vi "Main Page.vi"(8 "error in (no error)":errorcluster, 11 "Node Ptr":T1 format="%.0x") -> (0 "error out":errorcluster)   [LabVIEW 2015, in "Engine Simulation Toolkit System Explorer.lvlib"]
uses:
  Engine Simulation Toolkit System Explorer.lvlib
  <vilib>/NI Veristand/Custom Device API/Custom Device Item Ref.ctl
  Listbox State.ctl
  Main Page refnums.ctl
  Shared/Properties.vi
  <vilib>/NI Veristand/Custom Device API/Set Item Property (Boolean).vi
  <vilib>/NI Veristand/Custom Device API/Get Item Property (I32).vi
  <vilib>/NI Veristand/Custom Device API/Get Item Property (String Array).vi
  <vilib>/NI Veristand/Custom Device API/Get Item Property (Dependent File).vi
  <vilib>/NI Veristand/Custom Device API/Get Item Property (String).vi
  <vilib>/NI Veristand/Custom Device API/Set Item Property (I32).vi
  Shared/Constants and GUIDs.vi
  <userlib>/_OpenG.lib/array/array.llb/Delete Elements from 2D Array (String)__ogtk.vi
  <userlib>/_OpenG.lib/array/array.llb/Index 2D Array Elements (String)__ogtk.vi
  <vilib>/NI VeriStand/Custom Device API/Custom Device API.lvlib
  Shared/Engine Simulation Toolkit Shared.lvlib
  <vilib>/NI VeriStand/Custom Device Tools/Custom Device Utility Library/Custom Device Utility Library.lvlib
panel:
  in  "Reload bitfile":bool
  in  "Set master":bool
  in  "Remove bitfile":bool
  in  "Add bitfile":bool
  in  "Bitfile listbox":i32[](listbox) caption="Available APUs"
  in  "Header 3":cluster{"Section Name":string}={"Section Name"="Bitfile Selection"}
  in  "Remove APU":bool
  in  "Add APU":bool
  in  "APU listbox":i32[](listbox) caption="Available APUs"
  in  "Header 2":cluster{"Section Name":string}={"Section Name"="Available APUs"}
  in  "CPU":i32=-2
  in  "Rate decimation":i32=1 min=1
  in  "Execution priority":enum16{"Low", "Medium", "High"}(ring)=enum."Medium"
  out "CD Version":string caption="Custom device version"
  in  "Header":cluster{"Section Name":string}={"Section Name"="Engine Simulation Toolkit Settings"}
  in  "Name":string
  # "(-2: automatic)"
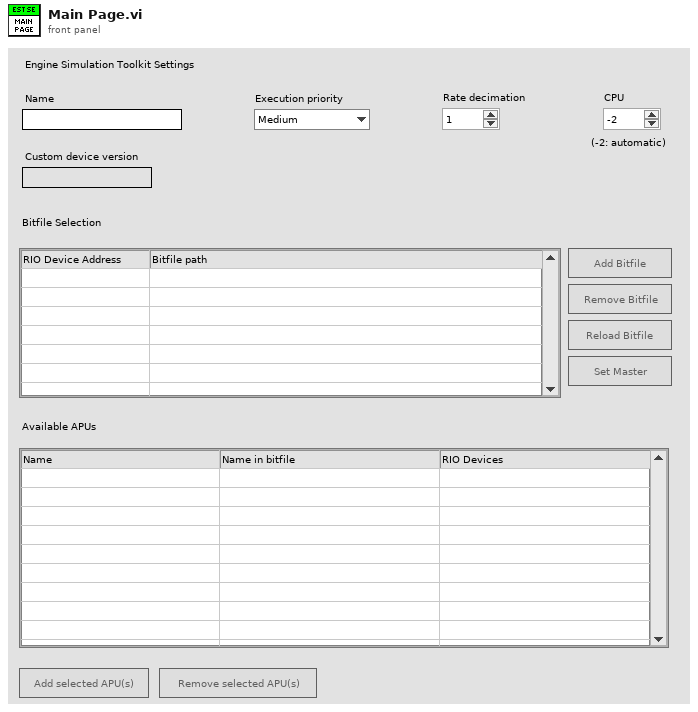
[diagram p1: front panel]
types:
  T1 = typedef "Custom Device API.lvlib/Custom Device Item Ref.ctl" = u64
  T2 = typedef "Engine Simulation Toolkit System Explorer.lvlib/Main Page refnums.ctl" = cluster{"Bitfile control refnums":cluster{"Add bitfile":refnum<vi>, "Remove bitfile":refnum<vi>, "Reload bitfile":refnum<vi>, "Set master":refnum<vi>, "Bitfile listbox":refnum<vi>}, "APU control refnums":cluster{"Add APU":refnum<vi>, "Remove APU":refnum<vi>, "APU listbox":refnum<vi>}}
  T3 = typedef "Engine Simulation Toolkit System Explorer.lvlib/Listbox State.ctl" = cluster{"listbox text":string[][], "not present item indexes":i32[], "selected values":i32[]}
  T4 = typedef "Custom Device API.lvlib/Custom Device Timed Loop Priority.ctl" = enum32{"Low", "Medium", "High"}
  T5 = typedef "Custom Device API.lvlib/Custom Device Item Info.ctl" = cluster{"Name":string, "Is Channel":bool, "GUID":string, "Is Waveform":bool}
  T6 = typedef "Custom Device API.lvlib/Custom Device Commands.ctl" = enum16{"Default", "Item renamed", "Shutdown", "Dynamic button pressed"}
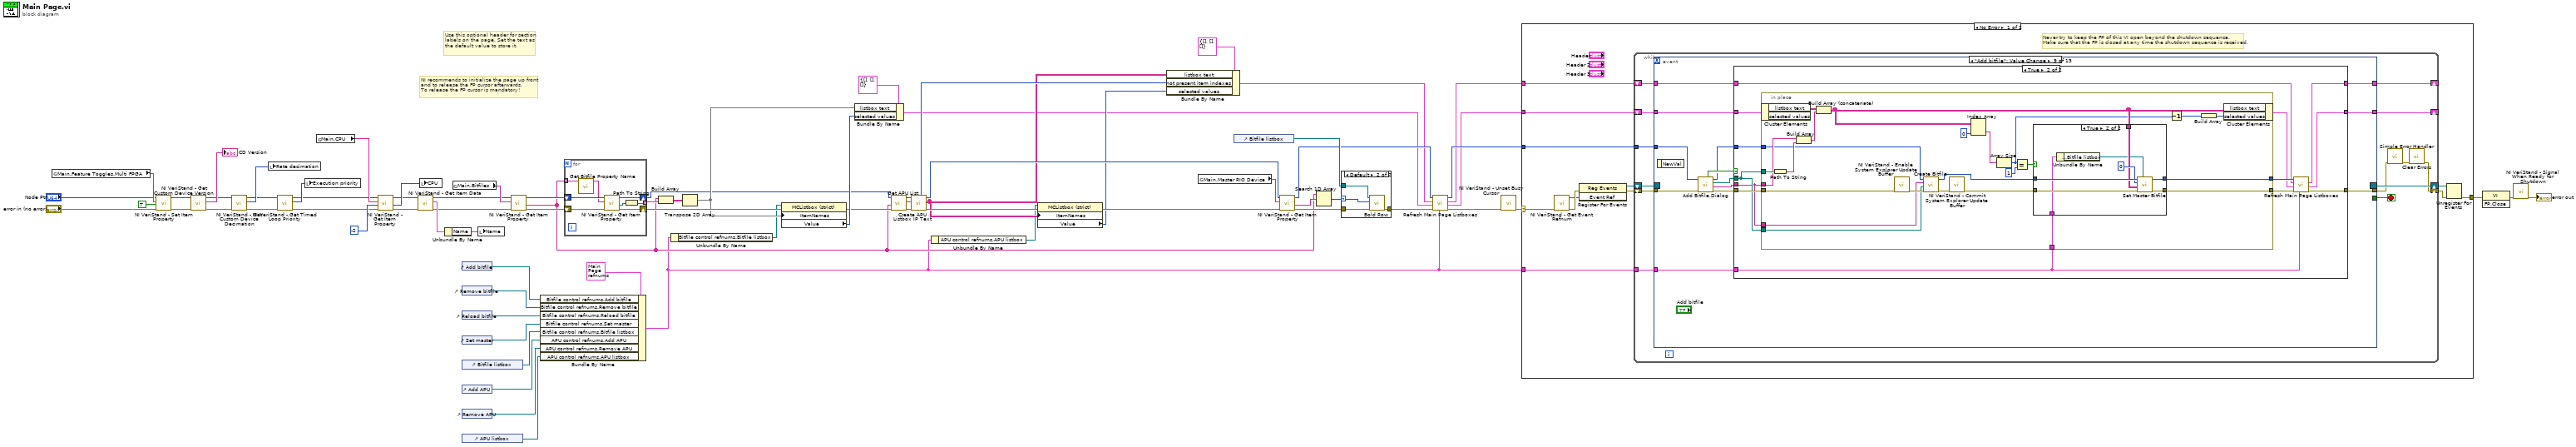
[diagram p0: block diagram]
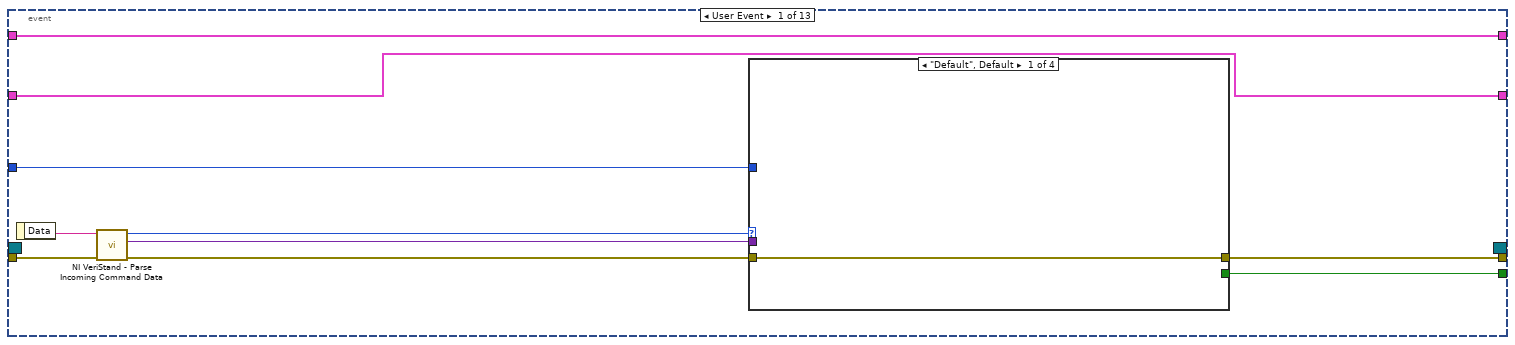
[diagram p3: hidden frame]
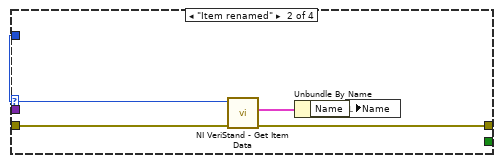
[diagram p4: hidden frame]
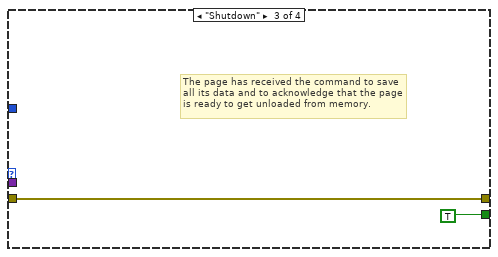
[diagram p5: hidden frame]
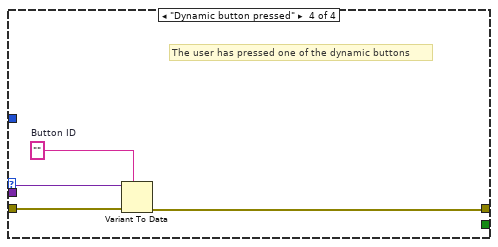
[diagram p6: hidden frame]
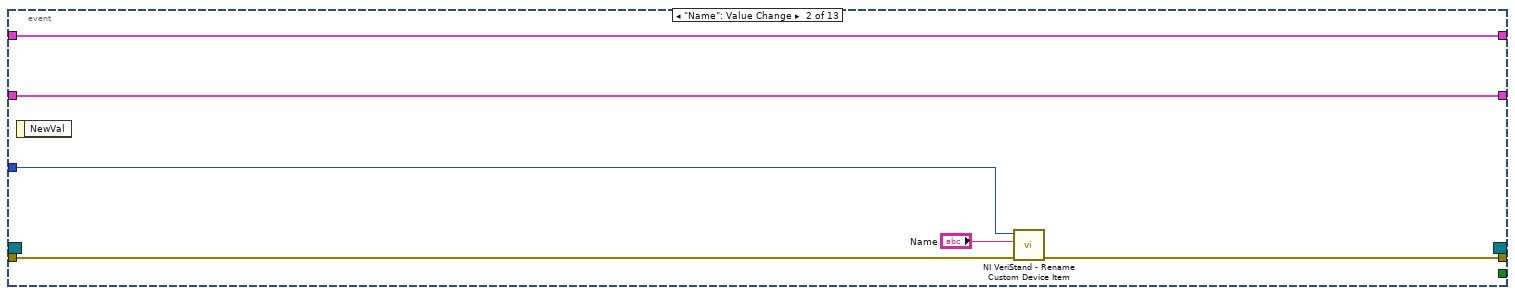
[diagram p7: hidden frame]
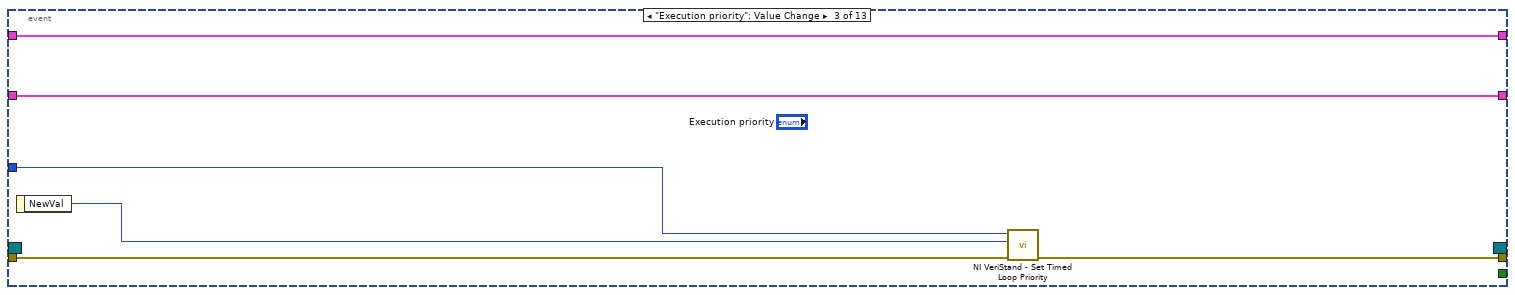
[diagram p8: hidden frame]
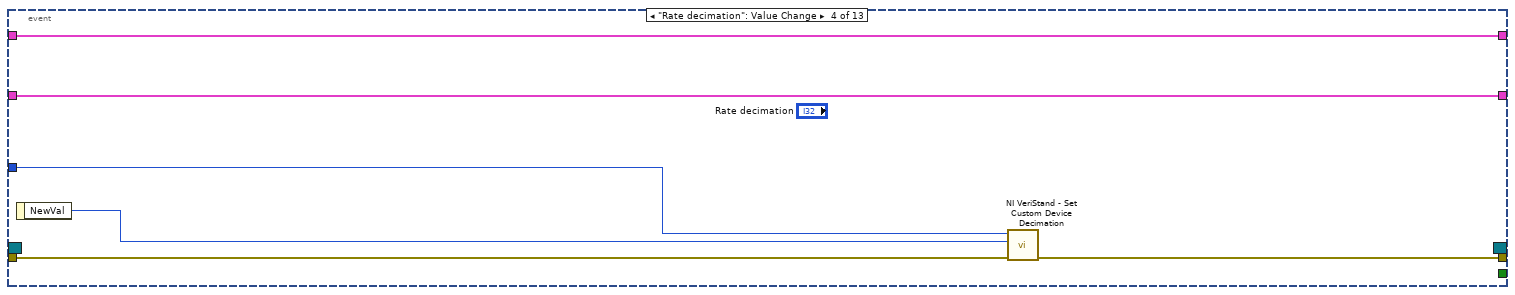
[diagram p9: hidden frame]
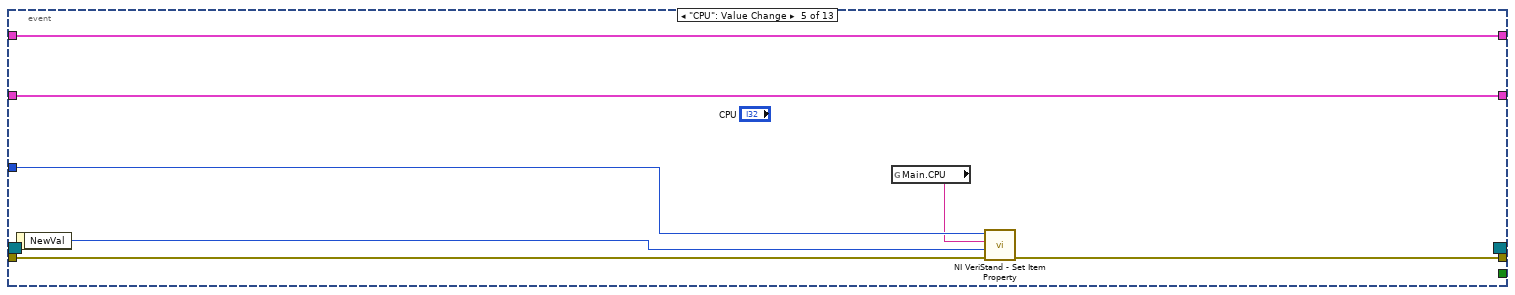
[diagram p10: hidden frame]
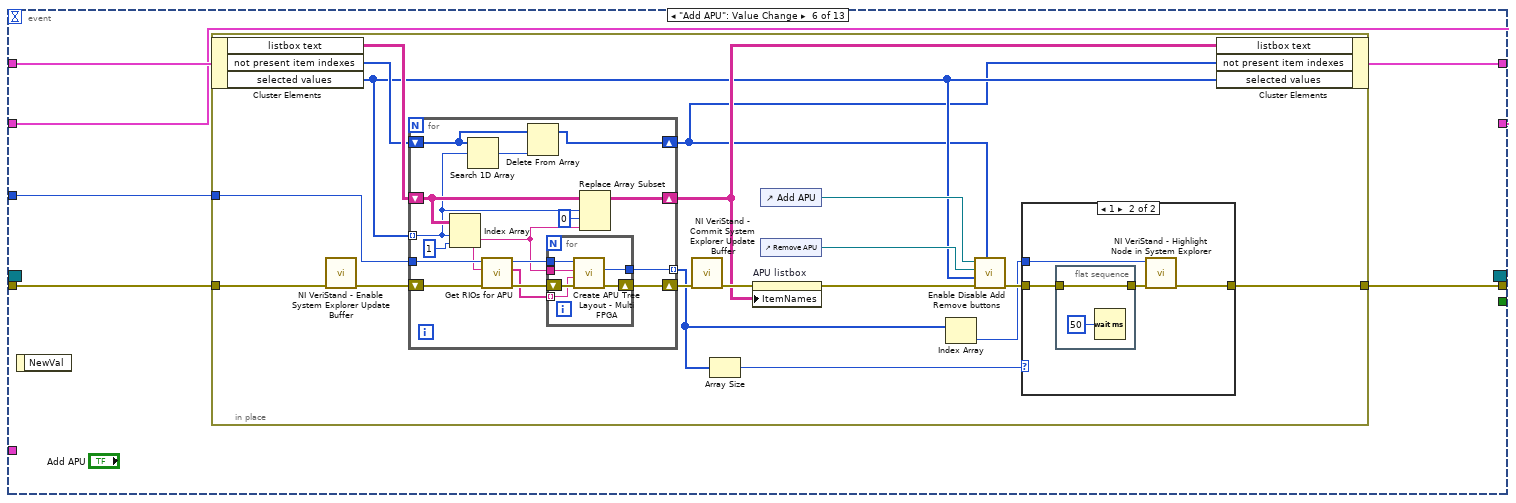
[diagram p11: hidden frame]
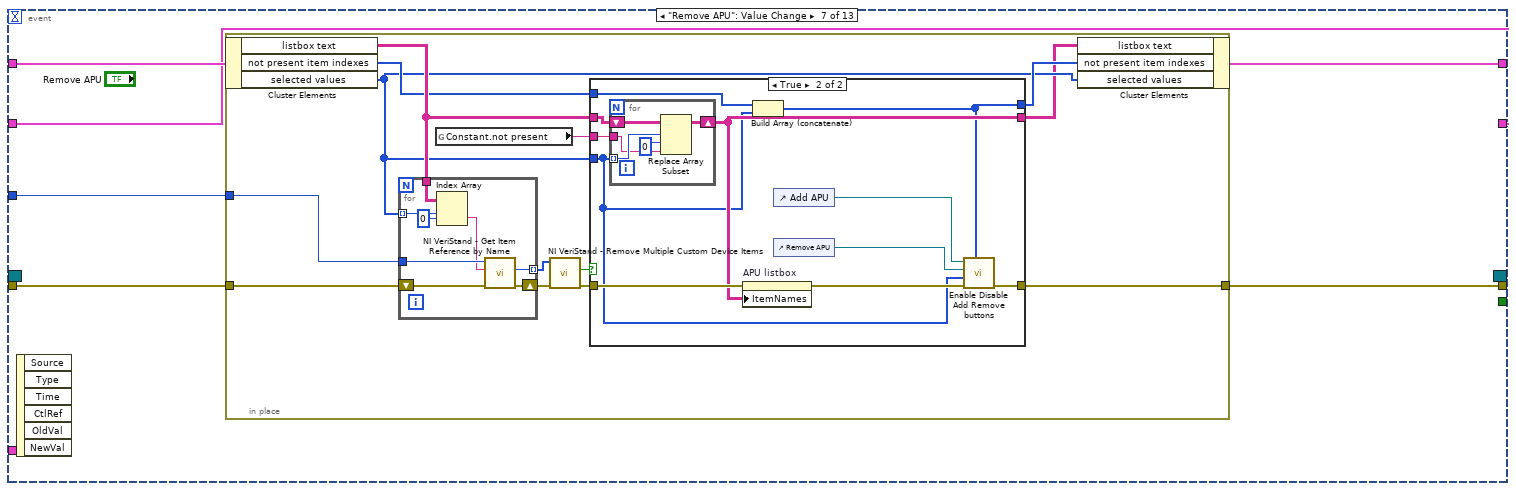
[diagram p13: hidden frame]
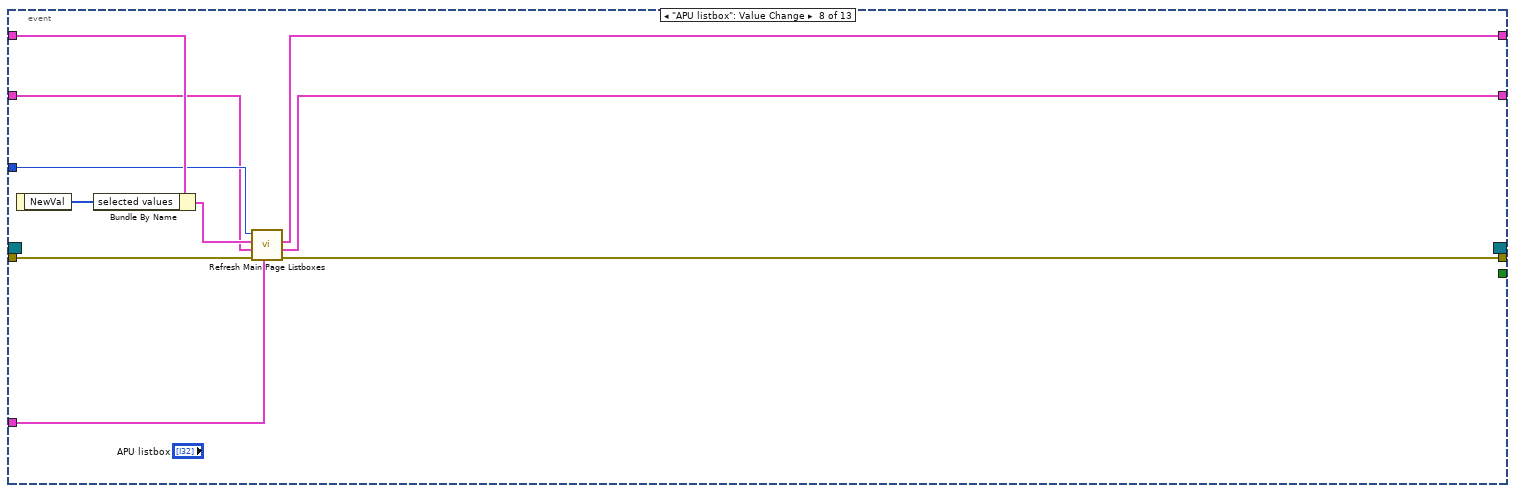
[diagram p15: hidden frame]
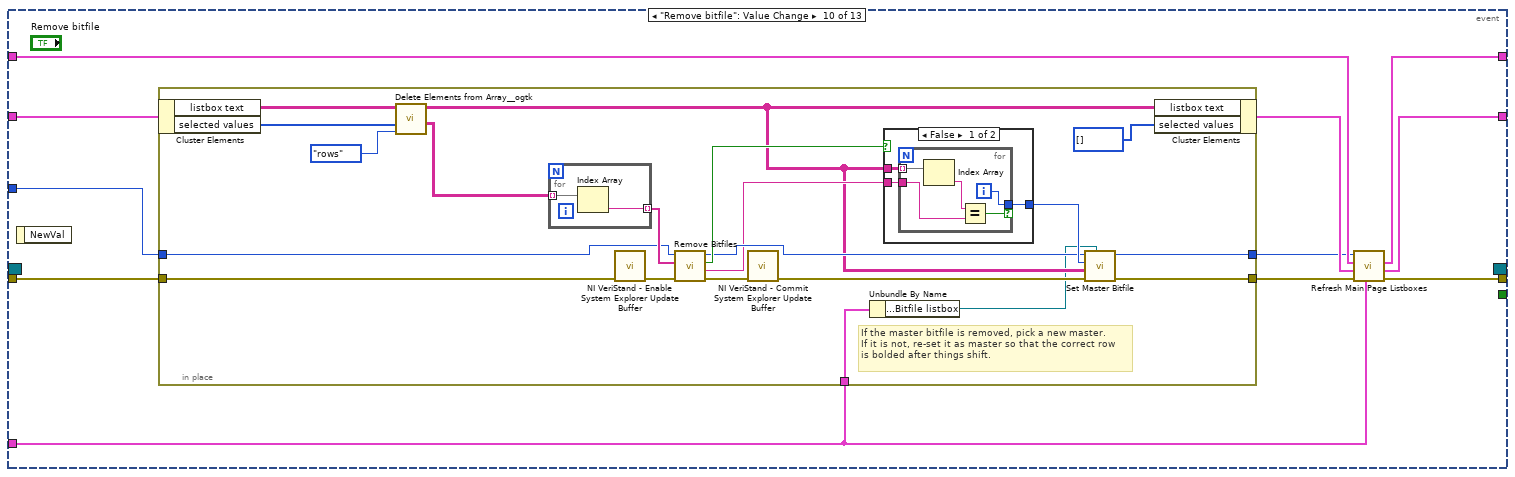
[diagram p18: hidden frame]
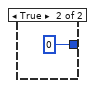
[diagram p19: hidden frame]
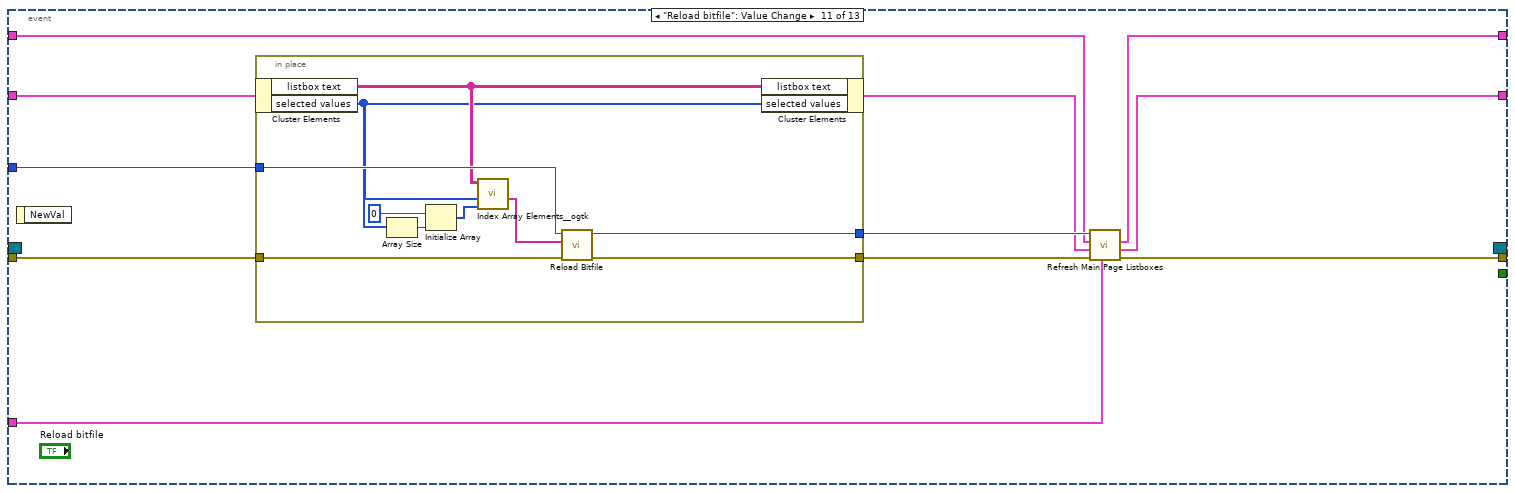
[diagram p20: hidden frame]
diagram:
  # "Use this optional header for section labels on the page. Set the text as the default value to store it."
  # "NI recommends to initialize the page up front\nand to release the FP cursor afterwards.\nTo release the FP cursor is mandatory!"
  n1 = global read "Properties.vi" "Main.Feature Toggles.Multi FPGA"() -> (w26:string)
  n2 = call-poly <vilib>:"NI VeriStand - Set Item Property.vi"("error in (no error)"="error in (no error)", "Value"=TRUE, "Property Name"=w26, "Item Ref in"="Node Ptr") -> ("error out"=w24:errorcluster, "Item Ref out"=w23:T1)  [unwired: 5 in, 1 out]
  n3 = call <vilib>:"NI VeriStand - Get Custom Device Version.vi"("error in (no error)"=w24, "Device Ref in"=w23) -> ("error out"=w69:errorcluster, "Value"=→"CD Version":string, "Device Ref out"=w66:T1)  [unwired: 7 in]
  n4 = call <vilib>:"NI VeriStand - Get Custom Device Decimation.vi"("error in (no error)"=w69, "Device Ref in"=w66) -> ("error out"=w67:errorcluster, "Decimation"=w65:i32, "Device Ref out"=w64:T1)  [unwired: 7 in]
  n5 = local write "Rate decimation"(w65) -> ()
  n6 = call <vilib>:"NI VeriStand - Get Timed Loop Priority.vi"("error in (no error)"=w67, "Device Ref in"=w64) -> ("error out"=w29:errorcluster, "Priority"=w63:T4, "Device Ref out"=w30:T1)  [unwired: 7 in]
  n7 = local write "Execution priority"(w63) -> ()
  n8 = global read "Properties.vi" "Main.CPU"() -> (w62:string)
  n9 = call-poly <vilib>:"NI VeriStand - Get Item Property.vi"("error in (no error)"=w29, "Default Value"=-2, "Property Name"=w62, "Item Ref in"=w30) -> ("error out"=w32:errorcluster, "Value"=w60:i32, "Item Ref out"=w33:T1)  [unwired: 4 in, 1 out]
  n10 = call <vilib>:"NI VeriStand - Get Item Data.vi"("error in (no error)"=w32, "Item Ref in"=w33) -> ("error out"=w38:errorcluster, "Item Info"=w71:T5, "Item Ref out"=w39:T1)  [unwired: 7 out]
  n11 = local write "CPU"(w60) -> ()
  n12 = Unbundle By Name(w71) -> ("Name"=w70:string)
  n13 = global read "Properties.vi" "Main.Bitfiles"() -> (w51:string)
  n14 = control-ref of="Add bitfile"() -> (w19:refnum<vi>)
  n15 = control-ref of="Remove bitfile"() -> (w18:refnum<vi>)
  n16 = control-ref of="Reload bitfile"() -> (w17:refnum<vi>)
  n17 = control-ref of="Set master"() -> (w16:refnum<vi>)
  n18 = control-ref of="Bitfile listbox"() -> (w13:refnum<vi>)
  n19 = control-ref of="Add APU"() -> (w15:refnum<vi>)
  n20 = control-ref of="Remove APU"() -> (w14:refnum<vi>)
  n21 = control-ref of="APU listbox"() -> (w12:refnum<vi>)
  n22 = local write "Name"(w70) -> ()
  n23 = call-poly <vilib>:"NI VeriStand - Get Item Property.vi"("error in (no error)"=w38, "Property Name"=w51, "Item Ref in"=w39) -> ("error out"=w50:errorcluster, "Value"=w31:string[], "Item Ref out"=w48:T1)  [unwired: 5 in, 1 out]
  n24 = Bundle By Name(cluster=T2 {"Bitfile control refnums"={"Add bitfile"=refnum, "Remove bitfile"=refnum, "Reload bitfile"=refnum, "Set master"=refnum, "Bitfile listbox"=refnum}, "APU control refnums"={"Add APU"=refnum, "Remove APU"=refnum, "APU listbox"=refnum}} ("Main Page refnums"), "Bitfile control refnums.Add bitfile"=w19, "Bitfile control refnums.Remove bitfile"=w18, "Bitfile control refnums.Reload bitfile"=w17, "Bitfile control refnums.Set master"=w16, "Bitfile control refnums.Bitfile listbox"=w13, "APU control refnums.Add APU"=w15, "APU control refnums.Remove APU"=w14, "APU control refnums.APU listbox"=w12) -> (w1:T2)
  n25 = for {
    shift-right: [w82] -> w49
    shift-left: w50 -> [w83]
    tunnel: [w78] -> w47 mode=indexing
    shift-right: [w80] -> w36
    shift-left: w48 -> [w81]
    tunnel: w31 -> [w76] mode=indexing
    n26 = call "Get Bitfile Property Name.vi"("RIO Device Address in"=w76) -> ("Bitfile Property Name"=w77:string)  [unwired: 10 in]
    n27 = call-poly <vilib>:"NI VeriStand - Get Item Property.vi"("error in (no error)"=w83, "Property Name"=w77, "Item Ref in"=w81) -> ("error out"=w82:errorcluster, "Path"=w79:path, "Item Ref out"=w80:T1)  [unwired: 4 in, 2 out]
    n28 = Path To String(path=w79) -> (string=w78:string)
  }
  n29 = Build Array(w31, w47) -> (w46:string[][])
  n30 = Unbundle By Name(w1) -> ("Bitfile control refnums.Bitfile listbox"=w11:refnum<vi>)
  n31 = Transpose 2D Array(2D array=w46) -> (transposed array=w45:string[][])
  n32 = property on="Property Node" class="MCListbox (strict)"(reference=w11, error in=w49, "ItemNames"=w45) -> (error out=w37:errorcluster, "Value"=w52:i32[])  [unwired: 1 out]
  n33 = Bundle By Name(cluster=T3 {"listbox text"=[], "not present item indexes"=[], "selected values"=[]} ("output cluster"), "listbox text"=w45, "selected values"=w52) -> (w3:T3)
  n34 = call "Get APU List.vi"("error in (no error)"=w37, "rio names"=w31, "Item Ref in"=w36) -> ("error out"=w59:errorcluster, "ips available"=w57:string[], "Item Ref out"=w58:T1)  [unwired: 6 in]
  n35 = call "Create APU Listbox IP Text.vi"("error in (no error)"=w59, "ips available"=w57, "Section Ref in"=w58) -> ("error out"=w56:errorcluster, "listbox text"=w28:string[][], "Section Ref out"=w35:T1, "not present item indexes"=w54:i32[])  [unwired: 5 in]
  n36 = Unbundle By Name(w1) -> ("APU control refnums.APU listbox"=w10:refnum<vi>)
  n37 = property on="Property Node" class="MCListbox (strict)"(reference=w10, error in=w56, "ItemNames"=w28) -> (error out=w55:errorcluster, "Value"=w27:i32[])  [unwired: 1 out]
  n38 = Bundle By Name(cluster=T3 {"listbox text"=[], "not present item indexes"=[], "selected values"=[]} ("output cluster"), "listbox text"=w28, "not present item indexes"=w54, "selected values"=w27) -> (w5:T3)
  n39 = global read "Properties.vi" "Main.Master RIO Device"() -> (w42:string)
  n40 = control-ref of="Bitfile listbox"() -> (w44:refnum<vi>)
  n41 = call-poly <vilib>:"NI VeriStand - Get Item Property.vi"("error in (no error)"=w55, "Property Name"=w42, "Item Ref in"=w35) -> ("error out"=w43:errorcluster, "Value"=w41:string, "Item Ref out"=w7:T1)  [unwired: 5 in, 1 out]
  n42 = Search 1D Array(1D array=w31, element=w41) -> (index of element=w40:i32)  [unwired: 1 in]
  n43 = case shown="Default" w40 {
    selector: w40 -> [_ w85]
    tunnel: w44 -> [_ w88]
    tunnel: [w84 w87] -> w9
    tunnel: w43 -> [w84 w86]
    frame -1 {
    }
    frame Default {
      n44 = call "Bold Row.vi"("error in (no error)"=w86, "Row (-2 : all)"=w85, "MulticolumnListbox in"=w88) -> ("error out"=w87:errorcluster)  [unwired: 7 in, 1 out]
    }
  }
  n45 = call "Refresh Main Page Listboxes.vi"("Main Page refnums"=w1, "error in (no error)"=w9, "bitfile listbox"=w3, "APU listbox"=w5, "Item Ref in"=w7) -> ("error out"=w8:errorcluster, "bitfile listbox out"=w2:T3, "APU listbox out"=w4:T3, "Item Ref out"=w6:T1)  [unwired: 3 in]
  n46 = call <vilib>:"NI VeriStand - Unset Busy Cursor.vi"("error in (no error)"=w8) -> ("error out"=w72:errorcluster)  [unwired: 10 out]
  n47 = case shown="No Error" w72 {
    selector: w72 -> [w92 w422]
    tunnel: [w97 w420] -> w75
    tunnel: w6 -> [w93 _]
    tunnel: w4 -> [w91 _]
    tunnel: w2 -> [w90 _]
    tunnel: w1 -> [w89 _]
    frame No Error {
      # "Never try to keep the FP of this VI open beyond the shutdown sequence.\nMake sure that the FP is closed at any time the shutdown sequence is received."
      n48 = call <vilib>:"NI VeriStand - Get Event Refnum.vi"("error in (no error)"=w92) -> ("error out"=w100:errorcluster, "Event Ref"=w96:refnum<user-event>)  [unwired: 9 out]
      n49 = register-events(error in=w100, w96) -> (reference out=w94:refnum<event-registration>, error out=w95:errorcluster)  [unwired: 1 in]
      n50 = while {
        tunnel: w93 -> [w109]
        shift-right: [w106] -> w98
        shift-left: w95 -> [w112]
        shift-right: [w113] -> w99
        shift-left: w94 -> [w111]
        shift-right: [w104] -> _
        shift-left: w91 -> [w105]
        shift-right: [w102] -> _
        shift-left: w90 -> [w103]
        tunnel: w89 -> [w101]
        stop <- w110 stop-if-true
        n51 = event shown="[8] \"Add bitfile\": Value Change" {
          selector: w111 -> [_ _ _ _ _ _ _ _ _ _ _ _ _]
          dyn-events: [_ _ _ _ _ _ _ _ _ _ _ _ _] -> w113
          timeout: _ -> [_ _ _ _ _ _ _ _ _ _ _ _ _]
          tunnel: w112 -> [w123 w141 w147 w153 w160 w166 w219 w267 w279 w343 w384 w409 w417]
          tunnel: [w119 _ _ _ _ _ _ _ _ _ _ _ _] -> w110
          tunnel: [w118 w140 w145 w151 w156 w165 w218 w266 w282 w335 w381 w398 w416] -> w108
          tunnel: w109 -> [w117 w139 w146 w152 w159 w164 w217 w265 w274 w341 w383 w404 w415]
          tunnel: w105 -> [w115 w137 w143 w149 w155 w163 w216 w268 w272 w339 w379 w402 w414]
          tunnel: [w115 w137 w143 w149 w155 w162 w215 w263 w271 w338 w378 w400 w411] -> w104
          tunnel: w103 -> [w114 w136 w142 w148 w154 w161 w214 w262 w281 w342 w385 w401 w419]
          tunnel: [w114 w136 w142 w148 w154 w161 w214 w261 w280 w337 w377 w399 w412] -> w102
          tunnel: w101 -> [_ _ _ _ _ _ _ w260 w270 w333 w375 w397 w410]
          event User Event {
            n52 = event-data() -> ("Data"=w122:string)  [unwired: 1 out]
            n53 = call <vilib>:"NI VeriStand - Parse Incoming Command Data.vi"("error in (no error)"=w123, "Incoming data"=w122) -> ("error out"=w121:errorcluster, "Outgoing data"=w116:variant, "Action"=w120:T6)  [unwired: 7 out]
            n54 = case shown="\"Default\", Default" w120 {
              tunnel: w121 -> [w124 w129 w130 w135]
              tunnel: [_ _ TRUE _] -> w119
              tunnel: [w124 w126 w130 w132] -> w118
              tunnel: w117 -> [_ w128 _ _]
              tunnel: w116 -> [_ _ _ w134]
              frame "Default", Default {
              }
              frame "Item renamed" {
                n55 = call <vilib>:"NI VeriStand - Get Item Data.vi"("error in (no error)"=w129, "Item Ref in"=w128) -> ("error out"=w126:errorcluster, "Item Info"=w127:T5)  [unwired: 8 out]
                n56 = Unbundle By Name(w127) -> ("Name"=w125:string)
                n57 = local write "Name"(w125) -> ()
              }
              frame "Shutdown" {
                # "The page has received the command to save all its data and to acknowledge that the page is ready to get unloaded from memory."
              }
              frame "Dynamic button pressed" {
                w133 = ""  # Button ID
                # "The user has pressed one of the dynamic buttons"
                n58 = Variant To Data(error in=w135, type=w133, Variant=w134) -> (error out=w132:errorcluster)  [unwired: 1 out]
              }
            }
          }
          event "Name": Value Change {
            n59 = event-data() -> ()  [unwired: 2 out]
            n60 = call <vilib>:"NI VeriStand - Rename Custom Device Item.vi"("error in (no error)"=w141, "New Name"="Name", "Item Ref in"=w139) -> ("error out"=w140:errorcluster)  [unwired: 1 in, 7 out]
          }
          event "Execution priority": Value Change {
            n61 = event-data() -> ("NewVal"=w144:enum16{"Low", "Medium", "High"})  [unwired: 1 out]
            n62 = call <vilib>:"NI VeriStand - Set Timed Loop Priority.vi"("error in (no error)"=w147, "Priority"=w144, "Device Ref in"=w146) -> ("error out"=w145:errorcluster)  [unwired: 7 in, 1 out]
          }
          event "Rate decimation": Value Change {
            n63 = event-data() -> ("NewVal"=w150:i32)  [unwired: 1 out]
            n64 = call <vilib>:"NI VeriStand - Set Custom Device Decimation.vi"("error in (no error)"=w153, "Decimation"=w150, "Device Ref in"=w152) -> ("error out"=w151:errorcluster)  [unwired: 7 in, 1 out]
          }
          event "CPU": Value Change {
            n65 = event-data() -> ("NewVal"=w158:i32)  [unwired: 1 out]
            n66 = global read "Properties.vi" "Main.CPU"() -> (w157:string)
            n67 = call-poly <vilib>:"NI VeriStand - Set Item Property.vi"("error in (no error)"=w160, "Value"=w158, "Property Name"=w157, "Item Ref in"=w159) -> ("error out"=w156:errorcluster)  [unwired: 5 in, 2 out]
          }
          event "Add APU": Value Change {
            n68 = event-data() -> ()  [unwired: 2 out]
            n69 = in-place {
              in-place-border: w166 -> [w174]
              in-place-border: [w173] -> w165
              in-place-border: w164 -> [w172]
              n70 = in-place-cluster #1(w163) -> ("listbox text"=w171:string[][], "not present item indexes"=w170:i32[], "selected values"=w168:i32[])
              n71 = call <vilib>:"NI VeriStand - Enable System Explorer Update Buffer.vi"("error in (no error)"=w174) -> ("error out"=w179:errorcluster)  [unwired: 10 in]
              n72 = for {
                tunnel: w172 -> [w195]
                shift-right: [w207] -> w184
                shift-left: w179 -> [w194]
                tunnel: w168 -> [w202] mode=indexing
                shift-right: [w204] -> w169
                shift-left: w171 -> [w205]
                shift-right: [w199] -> w167
                shift-left: w170 -> [w201]
                tunnel: [w198] -> w177 mode=indexing
                n73 = Index Array(array=w205, index (row)=w202, index (col)=1 ("disabled index (col)")) -> (element=w192:string)
                n74 = Search 1D Array(1D array=w201, element=w202) -> (index of element=w200:i32)  [unwired: 1 in]
                n75 = call "Get RIOs for APU.vi"("error in (no error)"=w194, "APU name"=w192, "Item Ref in"=w195) -> ("error out"=w197:errorcluster, "RIO Addresses"=w193:string[], "Item Ref out"=w196:T1)  [unwired: 6 in]
                n76 = Delete From Array(array=w201, index=w200) -> (array with subset deleted=w199:i32[])  [unwired: 1 in, 1 out]
                n77 = for {
                  tunnel: w192 -> [w212]
                  shift-right: [w213] -> w207
                  shift-left: w197 -> [w210]
                  tunnel: w193 -> [w208] mode=indexing
                  tunnel: w196 -> [w209]
                  tunnel: [w211] -> w198
                  n78 = call "Create APU Tree Layout - Multi FPGA.vi"("error in (no error)"=w210, "rio name"=w208, "engine name"=w212, "Section Ptr"=w209) -> ("error out"=w213:errorcluster, "APU ref"=w211:T1)  [unwired: 5 in, 1 out]
                }
                n79 = Replace Array Subset(array=w205, new element=w192, index (row)=w202, index (col)=0 ("disabled index (col)")) -> (w204:string[][])
              }
              n80 = call <vilib>:"NI VeriStand - Commit System Explorer Update Buffer.vi"("error in (no error)"=w184) -> ("error out"=w178:errorcluster)  [unwired: 10 in]
              n81 = Array Size(array=w177) -> (size(s)=w175:i32)
              n82 = property on="APU listbox" class="MCListbox (strict)"(error in=w178, "ItemNames"=w169) -> (error out=w183:errorcluster)  [unwired: 1 in, 1 out]
              n83 = control-ref of="Add APU"() -> (w181:refnum<vi>)
              n84 = control-ref of="Remove APU"() -> (w180:refnum<vi>)
              n85 = Index Array(array=w177) -> (element=w176:T1)  [unwired: 1 in]
              n86 = call "Enable Disable Add Remove buttons.vi"("not present item indexes"=w167, "error in (no error)"=w183, "selected items"=w168, "remove button"=w180, "add button"=w181) -> ("error out"=w182:errorcluster)  [unwired: 6 in]
              n87 = case shown="1" w175 {
                tunnel: w182 -> [w185 w186]
                tunnel: [w185 w189] -> w173
                tunnel: w176 -> [_ w188]
                frame Default {
                }
                frame 1 {
                  n88 = flat-sequence {
                    tunnel: [w190] -> w187
                    tunnel: w186 -> [w190]
                    frame #0 {
                      n89 = Wait (ms)(milliseconds to wait=u32 50) -> ()  [unwired: 1 out]
                    }
                  }
                  n90 = call <vilib>:"NI VeriStand - Highlight Node in System Explorer.vi"("error in (no error)"=w187, "Item Ref in"=w188) -> ("error out"=w189:errorcluster)  [unwired: 8 in, 1 out]
                }
              }
              n91 = in-place-cluster #1("listbox text"=w169, "not present item indexes"=w167, "selected values"=w168) -> (w162:T3)
            }
          }
          event "Remove APU": Value Change {
            n92 = event-data() -> ()  [unwired: 7 out]
            n93 = in-place {
              in-place-border: w219 -> [w227]
              in-place-border: [w226] -> w218
              in-place-border: w217 -> [w225]
              n94 = in-place-cluster #2(w216) -> ("listbox text"=w224:string[][], "not present item indexes"=w222:i32[], "selected values"=w221:i32[])
              n95 = for {
                tunnel: w221 -> [w258] mode=indexing
                tunnel: w224 -> [w259]
                tunnel: w225 -> [w255]
                tunnel: [w252] -> w231 mode=indexing
                shift-right: [w254] -> w232
                shift-left: w227 -> [w256]
                n96 = Index Array(array=w259, index (row)=w258, index (col)=0 ("disabled index (col)")) -> (element=w253:string)
                n97 = call <vilib>:"NI VeriStand - Get Item Reference by Name.vi"("error in (no error)"=w256, "Item Name"=w253, "Parent Ref in"=w255) -> ("error out"=w254:errorcluster, "Item Ref"=w252:T1)  [unwired: 5 in, 2 out]
              }
              n98 = global read "Constants and GUIDs.vi" "Constant.not present"() -> (w228:string)
              n99 = call <vilib>:"NI VeriStand - Remove Multiple Custom Device Items.vi"("error in (no error)"=w232, "Item Refs in"=w231) -> ("error out"=w230:errorcluster, "Deleted?"=w229:bool)  [unwired: 8 in]
              n100 = case shown="True" w229 {
                tunnel: [w234 w245] -> w226
                tunnel: w230 -> [w234 w242]
                tunnel: w221 -> [_ w237]
                tunnel: w224 -> [w235 w241]
                tunnel: w228 -> [_ w240]
                tunnel: [w235 w239] -> w220
                tunnel: w222 -> [w233 w238]
                tunnel: [w233 w236] -> w223
                frame False {
                }
                frame True {
                  n101 = for {
                    tunnel: w237 -> [w249] mode=indexing
                    shift-right: [w250] -> w239
                    shift-left: w241 -> [w251]
                    tunnel: w240 -> [w247]
                    n102 = Replace Array Subset(array=w251, new element=w247, index (row)=w249, index (col)=0 ("disabled index (col)")) -> (w250:string[][])
                  }
                  n103 = property on="APU listbox" class="MCListbox (strict)"(error in=w242, "ItemNames"=w239) -> (error out=w246:errorcluster)  [unwired: 1 in, 1 out]
                  n104 = Build Array (concatenate)(w238, w237) -> (w236:i32[])
                  n105 = control-ref of="Add APU"() -> (w244:refnum<vi>)
                  n106 = control-ref of="Remove APU"() -> (w243:refnum<vi>)
                  n107 = call "Enable Disable Add Remove buttons.vi"("not present item indexes"=w236, "error in (no error)"=w246, "selected items"=w237, "remove button"=w243, "add button"=w244) -> ("error out"=w245:errorcluster)  [unwired: 6 in]
                }
              }
              n108 = in-place-cluster #2("listbox text"=w220, "not present item indexes"=w223, "selected values"=w221) -> (w215:T3)
            }
          }
          event "APU listbox": Value Change {
            n109 = event-data() -> ("NewVal"=w269:i32[])  [unwired: 1 out]
            n110 = Bundle By Name(cluster=w268, "selected values"=w269) -> (w264:T3)
            n111 = call "Refresh Main Page Listboxes.vi"("Main Page refnums"=w260, "error in (no error)"=w267, "bitfile listbox"=w262, "APU listbox"=w264, "Item Ref in"=w265) -> ("error out"=w266:errorcluster, "bitfile listbox out"=w261:T3, "APU listbox out"=w263:T3)  [unwired: 3 in, 1 out]
          }
          event "Add bitfile": Value Change {
            n112 = event-data() -> ()  [unwired: 2 out]
            n113 = call "Add Bitfile Dialog.vi"("error in (no error)"=w279, "Item Ref in"=w274) -> ("error out"=w277:errorcluster, "RIO Device Address out"=w276:string, "Bitfile Path out"=w278:path, "Item Ref out"=w273:T1, "OK?"=w275:bool)  [unwired: 5 in]
            n114 = case shown="True" w275 {
              tunnel: w277 -> [w284 w298]
              tunnel: [w284 w292] -> w282
              tunnel: w281 -> [w285 w297]
              tunnel: [w285 w287] -> w280
              tunnel: w278 -> [_ w295]
              tunnel: w276 -> [_ w294]
              tunnel: w273 -> [_ w296]
              tunnel: w272 -> [w283 w290]
              tunnel: [w283 w289] -> w271
              tunnel: w270 -> [_ w286]
              frame False {
              }
              frame True {
                n115 = in-place {
                  in-place-border: [w312] -> w293
                  in-place-border: w295 -> [w320]
                  in-place-border: w294 -> [w318]
                  in-place-border: w298 -> [w317]
                  in-place-border: w296 -> [w308]
                  in-place-border: w295 -> [w304]
                  in-place-border: w294 -> [w305]
                  in-place-border: [w303] -> w291
                  in-place-border: w286 -> [w302]
                  n116 = in-place-cluster #3(w297) -> ("listbox text"=w322:string[][])  [unwired: 1 out]
                  n117 = Path To String(path=w320) -> (string=w319:string)
                  n118 = Build Array(w318, w319) -> (w321:string[])
                  n119 = Build Array (concatenate)(w322, w321) -> (w311:string[][])
                  n120 = call <vilib>:"NI VeriStand - Enable System Explorer Update Buffer.vi"("error in (no error)"=w317) -> ("error out"=w309:errorcluster)  [unwired: 10 in]
                  n121 = call "Create Bitfile.vi"("error in (no error)"=w309, "Bitfile Path in"=w304, "RIO Device Address in"=w305, "Item Ref in"=w308) -> ("error out"=w310:errorcluster, "Item Ref out"=w307:T1)  [unwired: 5 in, 1 out]
                  n122 = call <vilib>:"NI VeriStand - Commit System Explorer Update Buffer.vi"("error in (no error)"=w310) -> ("error out"=w306:errorcluster)  [unwired: 10 in]
                  n123 = Index Array(array=w311, index (col)=0 ("disabled index (col)")) -> (element=w313:string[])  [unwired: 1 in]
                  n124 = Array Size(array=w313) -> (size(s)=w300:i32)
                  n125 = Equal?(x=w300, y=1) -> (x = y?=w314:bool)
                  n126 = case shown="True" w314 {
                    tunnel: [w323 w330] -> w312
                    tunnel: w306 -> [w323 w329]
                    tunnel: w307 -> [w324 w332]
                    tunnel: [w324 w331] -> w303
                    tunnel: w311 -> [_ w327]
                    tunnel: w302 -> [_ w326]
                    frame False {
                    }
                    frame True {
                      n127 = Unbundle By Name(w326) -> ("Bitfile control refnums.Bitfile listbox"=w325:refnum<vi>)
                      n128 = call "Set Master Bitfile.vi"("MulticolumnListbox in"=w325, "error in (no error)"=w329, "listbox text"=w327, "Selected Value"=0, "Item Ref in"=w332) -> ("error out"=w330:errorcluster, "Item Ref out"=w331:T1)  [unwired: 5 in]
                    }
                  }
                  n129 = Decrement(x=w300) -> (x-1=w299:i32)
                  n130 = Build Array(w299) -> (w301:i32[])
                  n131 = in-place-cluster #3("listbox text"=w311, "selected values"=w301) -> (w288:T3)
                }
                n132 = call "Refresh Main Page Listboxes.vi"("Main Page refnums"=w286, "error in (no error)"=w293, "bitfile listbox"=w288, "APU listbox"=w290, "Item Ref in"=w291) -> ("error out"=w292:errorcluster, "bitfile listbox out"=w287:T3, "APU listbox out"=w289:T3)  [unwired: 3 in, 1 out]
              }
            }
          }
          event "Remove bitfile": Value Change {
            n133 = event-data() -> ()  [unwired: 2 out]
            n134 = in-place {
              in-place-border: w343 -> [w358]
              in-place-border: w341 -> [w351]
              in-place-border: [w348] -> w340
              in-place-border: [w346] -> w334
              in-place-border: w333 -> [w345]
              # "If the master bitfile is removed, pick a new master.\nIf it is not, re-set it as master so that the correct row\nis bolded after things shift."
              n135 = in-place-cluster #4(w342) -> ("listbox text"=w363:string[][], "selected values"=w362:i32[])
              n136 = call-poly <userlib>:"Delete Elements from Array__ogtk.vi"("delete (rows or columns)"=enum16{"rows", "columns"}."rows", "indices"=w362, "array"=w363) -> ("deleted elements"=w356:string[][], "array w/ subset deleted"=w347:string[][])  [unwired: 7 in]
              n137 = for {
                tunnel: w356 -> [w365] mode=indexing
                tunnel: [w364] -> w354 mode=indexing
                n138 = Index Array(array=w365) -> (element=w364:string)  [unwired: 1 in]
              }
              n139 = call <vilib>:"NI VeriStand - Enable System Explorer Update Buffer.vi"("error in (no error)"=w358) -> ("error out"=w349:errorcluster)  [unwired: 10 in]
              n140 = call "Remove Bitfiles.vi"("error in (no error)"=w349, "RIO Addresses"=w354, "Item Ref in"=w351) -> ("error out"=w359:errorcluster, "Previous master"=w352:string, "Need to select a new master?"=w355:bool, "Item Ref out"=w353:T1)  [unwired: 5 in]
              n141 = call <vilib>:"NI VeriStand - Commit System Explorer Update Buffer.vi"("error in (no error)"=w359) -> ("error out"=w350:errorcluster)  [unwired: 10 in]
              n142 = Unbundle By Name(w345) -> ("Bitfile control refnums.Bitfile listbox"=w344:refnum<vi>)
              n143 = case shown="False" w355 {
                tunnel: [w366 0 ("Selected Value")] -> w360
                tunnel: w347 -> [w368 _]
                tunnel: w352 -> [w367 _]
                frame False {
                  n144 = for {
                    tunnel: w368 -> [w373] mode=indexing
                    tunnel: w367 -> [w371]
                    tunnel: [w370] -> w366 if=w369
                    i -> [w370]
                    n145 = Index Array(array=w373) -> (element=w372:string)  [unwired: 1 in]
                    n146 = Equal?(x=w372, y=w371) -> (x = y?=w369:bool)
                  }
                }
                frame True {
                }
              }
              n147 = call "Set Master Bitfile.vi"("MulticolumnListbox in"=w344, "error in (no error)"=w350, "listbox text"=w347, "Selected Value"=w360, "Item Ref in"=w353) -> ("error out"=w348:errorcluster, "Item Ref out"=w346:T1)  [unwired: 5 in]
              n148 = in-place-cluster #4("listbox text"=w347, "selected values"=i32[] []) -> (w336:T3)
            }
            n149 = call "Refresh Main Page Listboxes.vi"("Main Page refnums"=w333, "error in (no error)"=w340, "bitfile listbox"=w336, "APU listbox"=w339, "Item Ref in"=w334) -> ("error out"=w335:errorcluster, "bitfile listbox out"=w337:T3, "APU listbox out"=w338:T3)  [unwired: 3 in, 1 out]
          }
          event "Reload bitfile": Value Change {
            n150 = event-data() -> ()  [unwired: 2 out]
            n151 = in-place {
              in-place-border: w384 -> [w395]
              in-place-border: [w389] -> w382
              in-place-border: w383 -> [w394]
              in-place-border: [w386] -> w380
              n152 = in-place-cluster #5(w385) -> ("listbox text"=w388:string[][], "selected values"=w387:i32[])
              n153 = Array Size(array=w387) -> (size(s)=w393:i32)
              n154 = Initialize Array(0, w393) -> (w391:i32[])
              n155 = call-poly <userlib>:"Index Array Elements__ogtk.vi"("indices 1"=w391, "indices 0"=w387, "array"=w388) -> ("elements"=w390:string[])  [unwired: 8 in]
              n156 = call "Reload Bitfile.vi"("error in (no error)"=w395, "RIO Addresses (all)"=w390, "Node Ptr"=w394) -> ("error out"=w389:errorcluster, "Node Ptr out"=w386:T1)  [unwired: 7 in]
              n157 = in-place-cluster #5("listbox text"=w388, "selected values"=w387) -> (w376:T3)
            }
            n158 = call "Refresh Main Page Listboxes.vi"("Main Page refnums"=w375, "error in (no error)"=w382, "bitfile listbox"=w376, "APU listbox"=w379, "Item Ref in"=w380) -> ("error out"=w381:errorcluster, "bitfile listbox out"=w377:T3, "APU listbox out"=w378:T3)  [unwired: 3 in, 1 out]
          }
          event "Set master": Value Change {
            n159 = event-data() -> ()  [unwired: 2 out]
            n160 = Unbundle By Name(w401) -> ("listbox text"=w406:string[][], "selected values"=w407:i32[])
            n161 = Unbundle By Name(w397) -> ("Bitfile control refnums.Bitfile listbox"=w396:refnum<vi>)
            n162 = Index Array(array=w407) -> (element=w408:i32)  [unwired: 1 in]
            n163 = call "Set Master Bitfile.vi"("MulticolumnListbox in"=w396, "error in (no error)"=w409, "listbox text"=w406, "Selected Value"=w408, "Item Ref in"=w404) -> ("error out"=w405:errorcluster, "Item Ref out"=w403:T1)  [unwired: 5 in]
            n164 = call "Refresh Main Page Listboxes.vi"("Main Page refnums"=w397, "error in (no error)"=w405, "bitfile listbox"=w401, "APU listbox"=w402, "Item Ref in"=w403) -> ("error out"=w398:errorcluster, "bitfile listbox out"=w399:T3, "APU listbox out"=w400:T3)  [unwired: 3 in, 1 out]
          }
          event "Bitfile listbox": Value Change {
            n165 = event-data() -> ("NewVal"=w418:i32[])  [unwired: 1 out]
            n166 = Bundle By Name(cluster=w419, "selected values"=w418) -> (w413:T3)
            n167 = call "Refresh Main Page Listboxes.vi"("Main Page refnums"=w410, "error in (no error)"=w417, "bitfile listbox"=w413, "APU listbox"=w414, "Item Ref in"=w415) -> ("error out"=w416:errorcluster, "bitfile listbox out"=w412:T3, "APU listbox out"=w411:T3)  [unwired: 3 in, 1 out]
          }
        }
        n168 = call <vilib>:"Simple Error Handler.vi"("error in (no error)"=w108) -> ("error out"=w107:errorcluster)  [unwired: 1 in, 7 out]
        n169 = call <vilib>:"Clear Errors.vi"("error in (no error)"=w107) -> ("error out"=w106:errorcluster)  [unwired: 1 in, 5 out]
      }
      n170 = Unregister For Events(event registration refnum=w99, error in=w98) -> (error out=w97:errorcluster)
    }
    frame Error {
      n171 = call <vilib>:"Simple Error Handler.vi"("error in (no error)"=w422) -> ("error out"=w421:errorcluster)  [unwired: 1 in, 7 out]
      n172 = call <vilib>:"Clear Errors.vi"("error in (no error)"=w421) -> ("error out"=w420:errorcluster)  [unwired: 1 in, 5 out]
    }
  }
  n173 = invoke class="VI" method="FP.Close"(error in=w75) -> (error out=w74:errorcluster)  [unwired: 2 in, 2 out]
  n174 = call <vilib>:"NI VeriStand - Signal When Ready for Shutdown.vi"("error in (no error)"=w74) -> ("error out"=→"error out":errorcluster)  [unwired: 10 out]
